vi "Actor Core.vi"(8 "error in":errorcluster, 11 "Test Actor in":refnum<class "Example Actor.lvclass">) -> (0 "error out":errorcluster, 3 "Actor out":refnum<class "Actor.lvclass">)   [LabVIEW 2017, in "Example Actor.lvlib" / "Example Actor.lvclass"]
doc: "(<B>Filename</B>: Actor Framework.lvlib:Actor.lvclass:Actor Core.vi)\n\nReceives messages to the actor, reacts to them, and initiates any error handling that may shut the actor down.\n\nDescendant classes may override this VI to append parallel tasks for the actor to complete while it handles messages. Overrides use the Call Parent Method node."
uses:
  Example Actor.lvclass
  C:/Program Files (x86)/National Instruments/LabVIEW 2017/vi.lib/ActorFramework/Actor/Actor.lvclass
  <vilib>/ActorFramework/Actor/Actor.lvclass
  Example Actor.lvclass/Example Actor.ctl
  <vilib>/ActorFramework/Message Enqueuer/Message Enqueuer.lvclass/Message Enqueuer.ctl
  <vilib>/ActorFramework/Message Enqueuer/Enqueue.vi
  <vilib>/ActorFramework/Stop Msg/Stop Msg.lvclass
  C:/Program Files (x86)/National Instruments/LabVIEW 2017/vi.lib/ActorFramework/Message/Message.lvclass
  <vilib>/ActorFramework/Message Priority Queue/Priority Enqueue.vi
  <vilib>/ActorFramework/Message Enqueuer/Message Enqueuer.lvclass
  monitored-actor-core/Source/Monitored Actor/Monitored Actor/Monitored Actor.lvclass
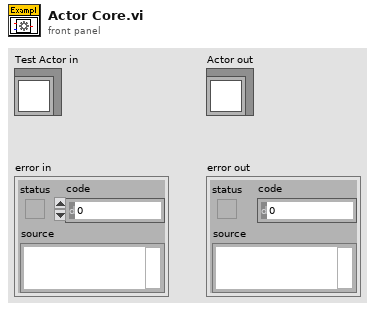
[diagram p1: front panel]
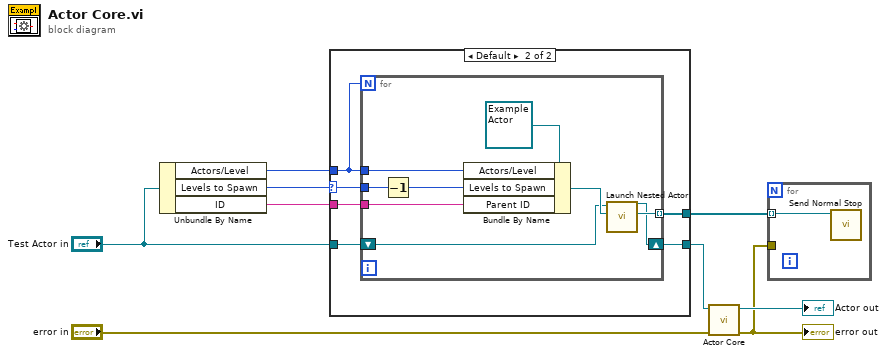
[diagram p0: block diagram]
diagram:
  n1 = Unbundle By Name("Test Actor in") -> ("Actors/Level"=w7:i32, "Levels to Spawn"=w1:i32, "ID"=w2:string)
  n2 = case shown="Default" w1 {
    selector: w1 -> [_ w12]
    tunnel: w7 -> [_ w11]
    tunnel: "Test Actor in" -> [w10 w16]
    tunnel: [w10 w15] -> w5
    tunnel: [_ w14] -> w4
    tunnel: w2 -> [_ w13]
    frame 0 {
    }
    frame Default {
      n3 = for {
        N: w11 -> [_]
        shift-right: [w17] -> w15
        shift-left: w16 -> [w18]
        tunnel: [w25] -> w14 mode=indexing
        tunnel: w13 -> [w23]
        tunnel: w12 -> [w22]
        tunnel: w11 -> [w20]
        n4 = Decrement(x=w22) -> (x-1=w21:i32)
        n5 = Bundle By Name(cluster=refnum<class "Example Actor.lvclass"> refnum ("Test Actor.lvclass"), "Actors/Level"=w20, "Levels to Spawn"=w21, "Parent ID"=w23) -> (w19:refnum<class "Example Actor.lvclass">)
        n6 = call <vilib>:"Launch Nested Actor.vi"("Nested Actor"=w19, "Caller Actor in"=w18) -> ("Nested Actor's Enqueuer"=w25:refnum<class "Message Enqueuer.lvclass">, "Caller Actor out"=w17:refnum<class "Example Actor.lvclass">)  [unwired: 7 in, 1 out]
      }
    }
  }
  n7 = call-parent "Actor Core.vi"("error in"="error in", "Actor in"=w5) -> ("error out"=w3:errorcluster, "Actor out"=→"Actor out":refnum<class "Actor.lvclass">)  [unwired: 8 in]
  "error out" <- w3
  n8 = for {
    tunnel: w4 -> [w26] mode=indexing
    tunnel: w3 -> [_]
    n9 = call <vilib>:"Send Normal Stop.vi"("Message Enqueuer"=w26) -> ()  [unwired: 10 in, 1 out]
  }
